vi "Calculate miniscan length.vi"(6 "Enum":enum16{"X", "Y"}(ring), 10 "XYZ Stop":cluster{"X":sgl, "Y":sgl, "Z":sgl}[](array[cluster]), 11 "XYZ Start":cluster{"X":sgl, "Y":sgl, "Z":sgl}[](array[cluster])) -> (2 "Number of pixels in single miniscan":i32, 3 "Number of pixels in each miniscan":i32[](array[numeric]))   [LabVIEW 2017]
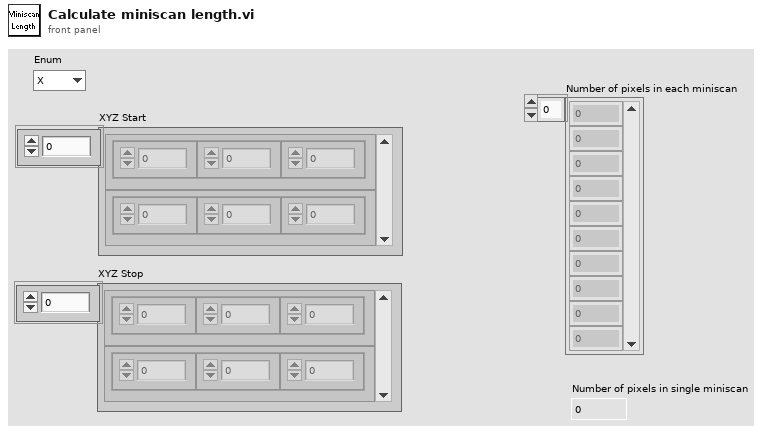
[diagram p1: front panel]
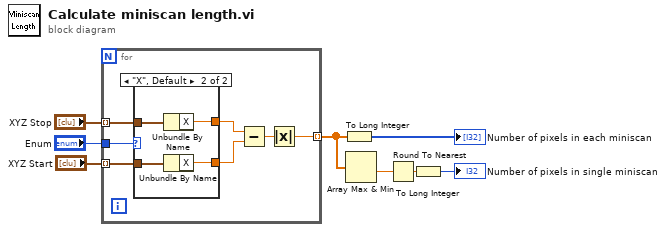
[diagram p0: block diagram]
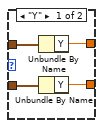
[diagram p2: hidden frame]
diagram:
  n1 = for {
    tunnel: [w14] -> w6 mode=indexing
    tunnel: "XYZ Start" -> [w13] mode=indexing
    tunnel: "XYZ Stop" -> [w12] mode=indexing
    tunnel: "Enum" -> [w9]
    n2 = case shown="\"X\", Default" w9 {
      tunnel: w13 -> [w19 w23]
      tunnel: w12 -> [w18 w22]
      tunnel: [w17 w21] -> w11
      tunnel: [w16 w20] -> w10
      frame "Y" {
        n3 = Unbundle By Name(w18) -> ("Y"=w17:sgl)
        n4 = Unbundle By Name(w19) -> ("Y"=w16:sgl)
      }
      frame "X", Default {
        n5 = Unbundle By Name(w22) -> ("X"=w21:sgl)
        n6 = Unbundle By Name(w23) -> ("X"=w20:sgl)
      }
    }
    n7 = Subtract(x=w11, y=w10) -> (x-y=w15:sgl)
    n8 = Absolute Value(x=w15) -> (abs(x)=w14:sgl)
  }
  n9 = To Long Integer(number=w6) -> (32bit integer=→"Number of pixels in each miniscan":i32[])
  n10 = Array Max & Min(array=w6) -> (min value=w7:sgl)  [unwired: 3 out]
  n11 = Round To Nearest(number=w7) -> (nearest integer value=w4:sgl)
  n12 = To Long Integer(number=w4) -> (32bit integer=→"Number of pixels in single miniscan":i32)
